vi "Update from Down.vi"(9 "Col":i32, 10 "Row":i32, 11 "Proto in":refnum<class "Heat Map.lvclass">) -> (3 "Proto out":refnum<class "Heat Map.lvclass">)   [LabVIEW 2021, in "Heat Map.lvclass"]
uses:
  Heat Map.lvclass
  Heat Map.lvclass/Heat Map.ctl
  Direction.ctl
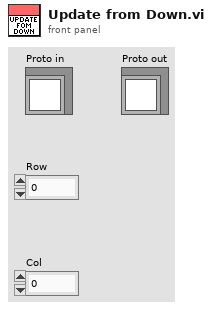
[diagram p1: front panel]
types:
  T1 = typedef "Heat Map.lvclass/Direction.ctl" = enum16{"Up", "Down", "Right", "Left"}
  T2 = map{cluster{"Row":i32, "Col":i32}, set{cluster{"Heat":i32, "Prev Steps":T1, "Step Count":i32}}}
  T3 = set{cluster{"Heat":i32, "Prev Steps":T1, "Step Count":i32}}
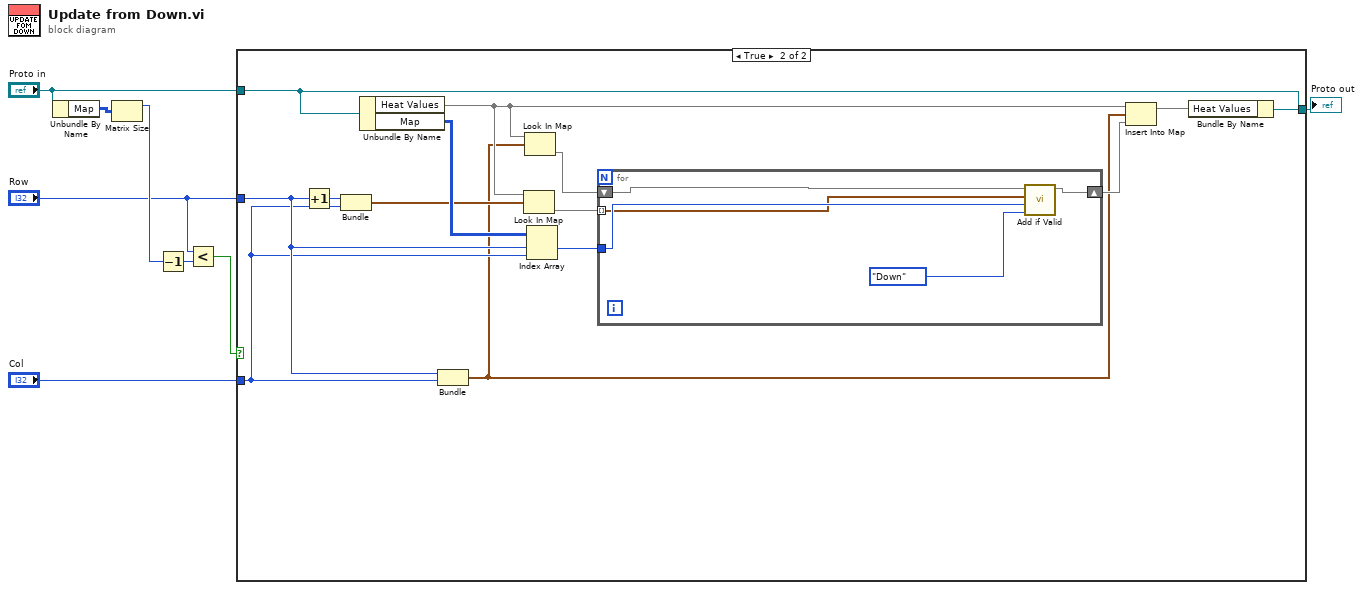
[diagram p0: block diagram]
diagram:
  n1 = Unbundle By Name("Proto in") -> ("Map"=w6:i32[][])
  n2 = Matrix Size(0:w6) -> (1:w2:i32)  [unwired: 1 out]
  n3 = Decrement(x=w2) -> (x-1=w4:i32)
  n4 = Less?(x="Row", y=w4) -> (x < y?=w5:bool)
  n5 = case shown="True" w5 {
    tunnel: [w9 w21] -> w8
    tunnel: "Proto in" -> [w9 w20]
    tunnel: "Row" -> [_ w17]
    tunnel: "Col" -> [_ w16]
    frame False {
    }
    frame True {
      n6 = Increment(x=w17) -> (x+1=w10:i32)
      n7 = Bundle(w10, "Col"=w16) -> (w19:cluster{i32, "Col":i32})  [unwired: 1 in]
      n8 = Unbundle By Name(w20) -> ("Heat Values"=w13:T2, "Map"=w23:i32[][])
      n9 = Bundle("Row"=w17, "Col"=w16) -> (w12:cluster{"Row":i32, "Col":i32})  [unwired: 1 in]
      n10 = Look In Map(map=w13, key=w19) -> (value=w15:T3)  [unwired: 1 in, 1 out]
      n11 = Look In Map(map=w13, key=w12) -> (value=w11:T3)  [unwired: 1 in, 1 out]
      n12 = Index Array(array=w23, index (row)=w17, index (col)=w16) -> (element=w18:i32)
      n13 = for {
        tunnel: w15 -> [w24] mode=indexing
        tunnel: w18 -> [w25]
        shift-right: [w28] -> w14
        shift-left: w11 -> [w27]
        n14 = call "Add if Valid.vi"("Direction"=Direction."Down" ("Dir"), "Heat"=w25, "element"=w24, "set"=w27) -> ("set"=w28:T3)  [unwired: 7 in]
      }
      n15 = Insert Into Map(map in=w13, key=w12, value=w14) -> (map out=w22:T2)  [unwired: 2 out]
      n16 = Bundle By Name(cluster=w20, "Heat Values"=w22) -> (w21:refnum<class "Heat Map.lvclass">)
    }
  }
  "Proto out" <- w8
